vi "TMP007 Read.vi"(7 "I2C Channel":u8, 8 "error in (no error)":errorcluster, 10 "I2C Slave Address":u8 format="%.0x", 11 "LINX Resource in":T2) -> (0 "error out":errorcluster, 1 "Conversion Time (S)":dbl format="%#_g s", 2 "Temp Readings":T1 {"Ambient Temp (°F)" format="%.2f °F"; "Ambient Temp (°C)" format="%.2f °C"; "Object Temp (°F)" format="%.2f °F"; "Object Temp (°C)" format="%.2f °C"}, 3 "LINX Resource":T2)   [LabVIEW 2014]
uses:
  <vilib>/MakerHub/LINX/Private/Type Defs/LINX Ref.ctl
  <vilib>/MakerHub/LINX/Private/Type Defs/Platform.ctl
  <vilib>/MakerHub/LINX/Private/Type Defs/Interface.ctl
  <vilib>/MakerHub/LINX/Private/Device/Type Defs/LINX Device Config.ctl
  <vilib>/MakerHub/LINX/Private/Device/Type Defs/TCP Config.ctl
  <vilib>/MakerHub/LINX/Private/Device/Type Defs/Channels.ctl
  <vilib>/MakerHub/LINX/Private/Local IO/LinxI2cWrite.vi
  <vilib>/MakerHub/LINX/Public/Utilities/Check Channel.vi
  <vilib>/myRIO/Instrument Drivers/Onboard IO/I2C/vis/Write.vi
  <vilib>/MakerHub/LINX/Private/Utilties/Generate Error.vi
  <vilib>/MakerHub/LINX/Private/Utilties/Channel FGVs/I2C Channels.vi
  <vilib>/Utility/error.llb/Error Cluster From Error Code.vi
  <vilib>/myRIO/Common/Instrument Driver Framework/myRIO v1.0/I2C/vis/myRIO v1.0 Write I2C.vi
  <vilib>/MakerHub/LINX/LMH-LINX.lvlib
  <vilib>/MakerHub/LINX/Private/Device/Device.lvlib
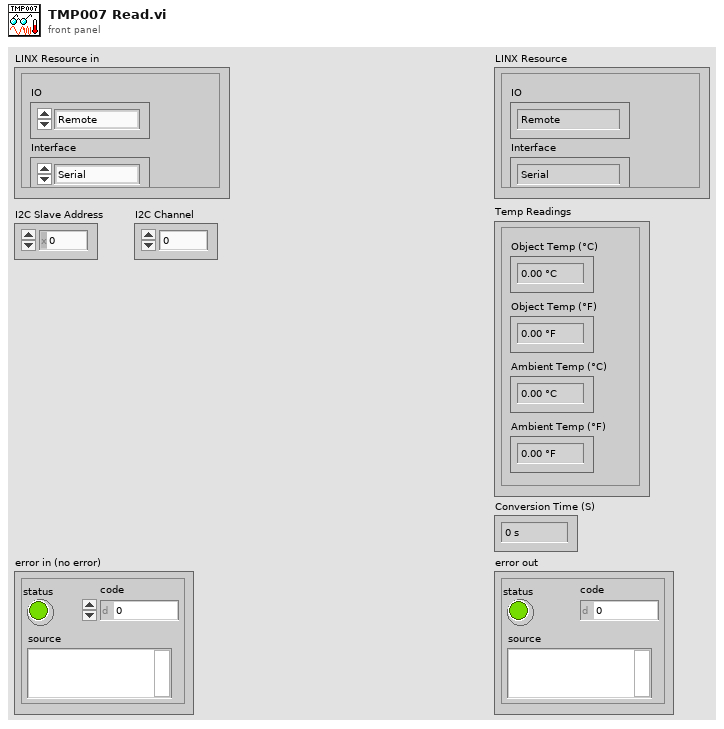
[diagram p1: front panel]
types:
  T1 = cluster{"Object Temp (°C)":dbl, "Object Temp (°F)":dbl, "Ambient Temp (°C)":dbl, "Ambient Temp (°F)":dbl}
  T2 = typedef "LMH-LINX.lvlib/LINX Ref.ctl" = cluster{"IO":T3, "Interface":T4, "LINX Device Config":T5}
  T3 = typedef "LMH-LINX.lvlib/Platform.ctl" = enum16{"Remote", "Local"}
  T4 = typedef "LMH-LINX.lvlib/Interface.ctl" = enum16{"Serial", "TCP"}
  T5 = typedef "LMH-LINX.lvlib/Device.lvlib/LINX Device Config.ctl" = cluster{"Interface":T4, "COM Port":refnum<visa-resource-name>, "TCP Configuration":T6, "Device Family":u8, "Device ID":u8, "Device Name":string, "TCP Ref":refnum<k5>, "Channels":T7}
  T6 = typedef "LMH-LINX.lvlib/Device.lvlib/TCP Config.ctl" = cluster{"IP Address":string, "Port":u16}
  T7 = typedef "LMH-LINX.lvlib/Channels.ctl" = cluster{"DI":u8[], "DO":u8[], "AI":u8[], "AO":u8[], "PWM":u8[], "QE":u8[], "UART":u8[], "I2C 2":u8[], "SPI":u8[], "CAN":u8[], "Servo":u8[], "AI Ref (V)":dbl, "AI Resolution (Bits)":u8, "AO Ref (V)":dbl, "AO Resolution (Bits)":u8}
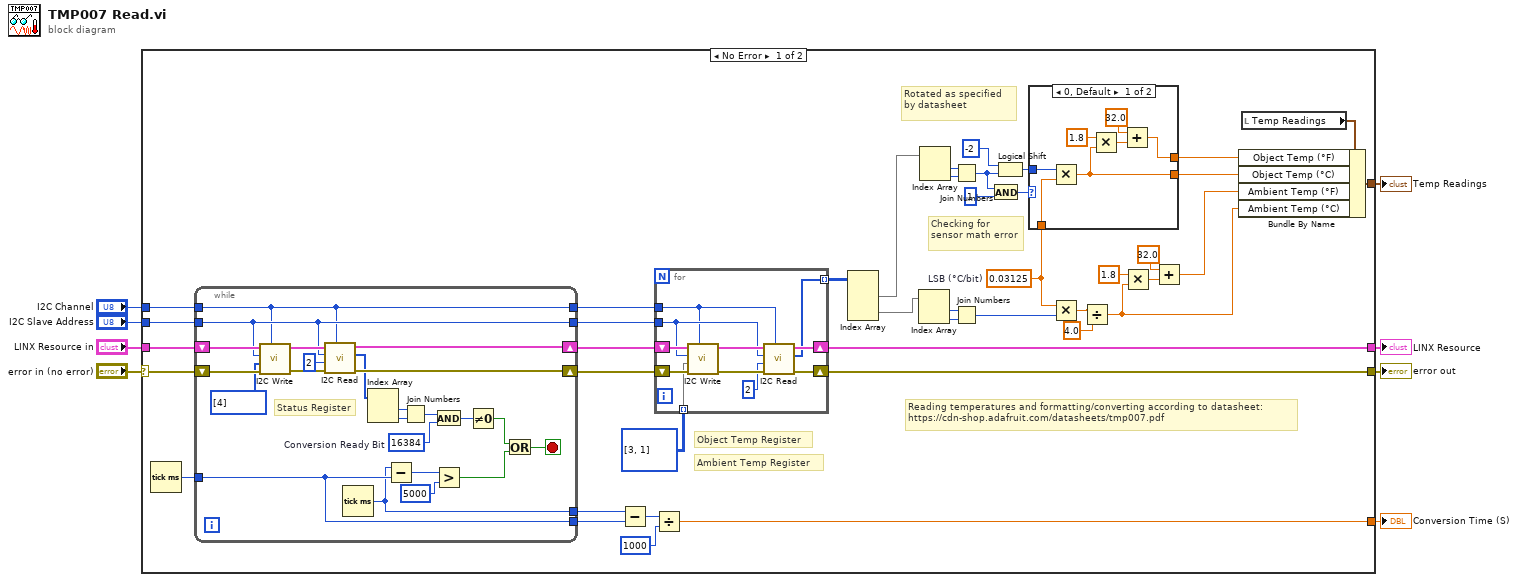
[diagram p0: block diagram]
diagram:
  n1 = case shown="No Error" "error in (no error)" {
    selector: "error in (no error)" -> [w9 w92]
    tunnel: [w50 w93] -> w8
    tunnel: [w49 w92] -> w7
    tunnel: [w26 _] -> w6
    tunnel: "LINX Resource in" -> [w25 w93]
    tunnel: "I2C Channel" -> [w22 _]
    tunnel: "I2C Slave Address" -> [w21 _]
    tunnel: [w14 _] -> w2
    frame No Error {
      w34 = 0.03125  # LSB (°C/bit)
      # "Reading temperatures and formatting/converting according to datasheet:\nhttps://cdn-shop.adafruit.com/datasheets/tmp007.pdf"
      # "Rotated as specified by datasheet"
      # "Checking for sensor math error"
      # "Ambient Temp Register"
      # "Object Temp Register"
      n2 = Tick Count (ms)() -> (millisecond timer value=w18:u32)
      n3 = while {
        tunnel: w22 -> [w65]
        tunnel: w21 -> [w66]
        tunnel: [w65] -> w20
        tunnel: [w66] -> w19
        shift-right: [w67] -> w24
        shift-left: w9 -> [w72]
        shift-right: [w68] -> w23
        shift-left: w25 -> [w73]
        tunnel: w18 -> [w52]
        tunnel: [w52] -> w17
        tunnel: [w51] -> w13
        stop <- w54 stop-if-true
        w59 = u16 16384  # Conversion Ready Bit
        # "Status Register"
        n4 = call <vilib>:"I2C Write.vi"("I2C Channel"=w65, "Error In"=w72, "Data"=u8[] [4], "I2C Slave Address (0)"=w66, "LINX Resource"=w73) -> ("Error Out"=w69:errorcluster, "LINX Resource"=w70:T2)  [unwired: 5 in]
        n5 = call <vilib>:"I2C Read.vi"("I2C Channel"=w65, "Error In"=w69, "Bytes To Read"=u8 2, "I2C Slave Address (0)"=w66, "LINX Resource"=w70) -> ("Error Out"=w67:errorcluster, "Data"=w62:u8[], "LINX Resource"=w68:T2)  [unwired: 4 in]
        n6 = Tick Count (ms)() -> (millisecond timer value=w51:u32)
        n7 = Index Array(array=w62) -> (element #1=w63:u8, element #2=w61:u8)  [unwired: 2 in]
        n8 = Subtract(x=w51, y=w52) -> (x-y=w58:u32)
        n9 = Join Numbers(hi=w63, lo=w61) -> ((hi.lo)=w60:u16)
        n10 = And(x=w60, y=w59) -> (x .and. y?=w56:u16)
        n11 = Greater?(x=w58, y=u32 5000) -> (0:w55:bool)
        n12 = Not Equal To 0?(x=w56) -> (x != 0?=w53:bool)
        n13 = Or(x=w53, y=w55) -> (x .or. y?=w54:bool)
      }
      n14 = Subtract(x=w13, y=w17) -> (x-y=w16:u32)
      n15 = Divide(x=w16, y=u32 1000) -> (x/y=w14:dbl)
      n16 = for {
        tunnel: w19 -> [w85]
        tunnel: w20 -> [w84]
        shift-right: [w86] -> w49
        shift-left: w24 -> [w91]
        shift-right: [w87] -> w50
        shift-left: w23 -> [w90]
        tunnel: u8[][] [[3], [1]] ("Data") -> [w82] mode=indexing
        tunnel: [w81] -> w47 mode=indexing
        n17 = call <vilib>:"I2C Write.vi"("I2C Channel"=w84, "Error In"=w91, "Data"=w82, "I2C Slave Address (0)"=w85, "LINX Resource"=w90) -> ("Error Out"=w88:errorcluster, "LINX Resource"=w89:T2)  [unwired: 5 in]
        n18 = call <vilib>:"I2C Read.vi"("I2C Channel"=w84, "Error In"=w88, "Bytes To Read"=u8 2, "I2C Slave Address (0)"=w85, "LINX Resource"=w89) -> ("Error Out"=w86:errorcluster, "Data"=w81:u8[], "LINX Resource"=w87:T2)  [unwired: 4 in]
      }
      n19 = Index Array(array=w47) -> (element #1=w46:u8[], element #2=w45:u8[])  [unwired: 4 in]
      n20 = Index Array(array=w45) -> (element #1=w42:u8, element #2=w41:u8)  [unwired: 2 in]
      n21 = Index Array(array=w46) -> (element #1=w43:u8, element #2=w44:u8)  [unwired: 2 in]
      n22 = Join Numbers(hi=w43, lo=w44) -> ((hi.lo)=w39:u16)
      n23 = Join Numbers(hi=w42, lo=w41) -> ((hi.lo)=w37:u16)
      n24 = And(x=w39, y=u16 1) -> (x .and. y?=w33:u16)
      n25 = Logical Shift(y=i16 -2, x=w39) -> (x << y=w35:u16)
      n26 = case shown="0, Default" w33 {
        tunnel: w35 -> [w80 _]
        tunnel: w34 -> [w79 _]
        tunnel: [w75 _] -> w32
        tunnel: [w74 _] -> w31
        frame 0, Default {
          n27 = Multiply(x=w80, y=w79) -> (x*y=w75:dbl)
          n28 = Multiply(x=1.8, y=w75) -> (x*y=w76:dbl)
          n29 = Add(x=32.0, y=w76) -> (x+y=w74:dbl)
        }
        frame 1 {
          # "Sensor math error found on sensor"
        }
      }
      n30 = Multiply(x=w34, y=w37) -> (x*y=w12:dbl)
      n31 = Divide(x=w12, y=4.0) -> (x/y=w11:dbl)
      n32 = Multiply(x=1.8, y=w11) -> (x*y=w30:dbl)
      n33 = Add(x=32.0, y=w30) -> (x+y=w27:dbl)
      n34 = local read "Temp Readings"() -> (w36:T1)
      n35 = Bundle By Name(cluster=w36, "Object Temp (°F)"=w31, "Object Temp (°C)"=w32, "Ambient Temp (°F)"=w27, "Ambient Temp (°C)"=w11) -> (w26:T1)
    }
    frame Error {
    }
  }
  "error out" <- w7
  "LINX Resource" <- w8
  "Temp Readings" <- w6
  "Conversion Time (S)" <- w2
